vi "FuncImg-Extract selected ROIs data-Core.vi"(9 "System Cluster":T7 {"ROI number" min=1 format="ROI %.0f"}, 10 "Input cluster":T3={"Channel A?"=FALSE, "MovCor enabled"=FALSE, "Cycle time-stamps (us)"=[], "Cycle length (us)"=0.0, "[Pixels in ROI]"=[], "Z-Stack Header data"={"Number of POI"=0, "Number of Miniscans"=0, "Number of Trials"=0, "Number of Cycles "=0, "# Averaged Frames"=0, "Laser power (%)"=0, "Pockels"=0.0, "Acquisition Length (sec)"=0.0, "Fill time (us)"=0.0, "DwellTime (us)"=0.0, "Miniscan Dwell time per pixel (us)"=0.0, "PMT 1"=0.0, "PMT 2"=0.0, "Back Apperture"=0.0, "Zoom"=0.0, "Number of Pixels in Miniscan"=0, "Frame Size"=200, "Field of View"=0.0, "X centre"=0.0, "Y centre"=0.0, "AOL Z"=0.0}, "[ROI Time (us)]"=[], "Path out"=path "", "Version index"=0} {"Z-Stack Header data"."Frame Size" items=["100X100"=100, "128X128"=128, "200X200"=200, "256X256"=256, "512X512"=512, "1024x1024"=1024, "2048x2048"=2048]; "Z-Stack Header data"."Back Apperture" format="%#.6g"; "Z-Stack Header data"."Pockels" format="%#.6g"; "Z-Stack Header data"."PMT 2" format="%#.6g"; "Z-Stack Header data"."PMT 1" format="%#.6g"; "Z-Stack Header data"."Miniscan Dwell time per pixel (us)" format="%#.6g"; "Z-Stack Header data"."Zoom" format="%#.6g"; "Z-Stack Header data"."DwellTime (us)" format="%#.6g"; "Z-Stack Header data"."Acquisition Length (sec)" format="%#.6g"; "Z-Stack Header data"."Fill time (us)" format="%#.6g"}) -> (0 "error IO":errorcluster, 1 "Points per trial":i32, 3 "Interface-Data format definition":T4)   [LabVIEW 2017]
uses:
  xcontrol/Interface VIs/Interface typedefs/Interface-ROI selection cluster.ctl
  Typedefs/ROI ID Enum.ctl
  xcontrol/Interface VIs/Interface typedefs/Interface-Data format definition.ctl
  xcontrol/Typedefs/Xctl-XY data type definition.ctl
  xcontrol/Typedefs/Xctrl-ROI type enum.ctl
  Experiment header interface/Typedefs/Header parameters cluster-Zstack.ctl
  Typedefs/Frame Size.ctl
  xcontrol/XGrapher.xctl
panel:
  # "<--- Timeline data already decimated\n          for memory efficiency."
  # "Zstack header parameters"
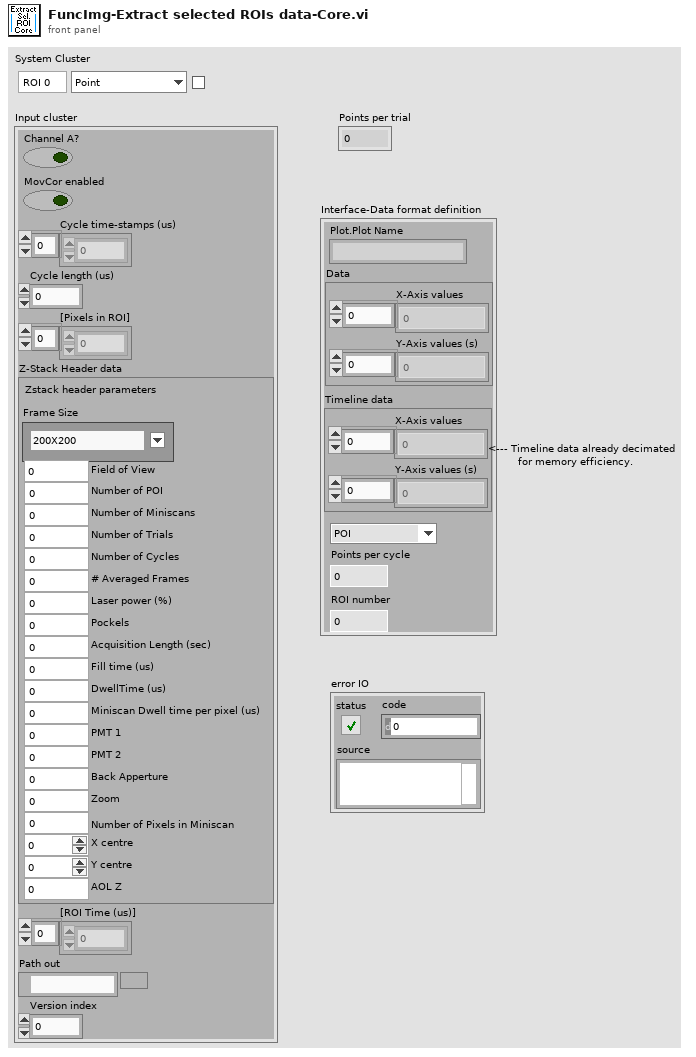
[diagram p1: front panel]
types:
  T1 = typedef "Header parameters cluster-Zstack.ctl" = cluster{"Number of POI":u16, "Number of Miniscans":u16, "Number of Trials":u16, "Number of Cycles ":u16, "# Averaged Frames":u16, "Laser power (%)":u8, "Pockels":dbl, "Acquisition Length (sec)":dbl, "Fill time (us)":dbl, "DwellTime (us)":dbl, "Miniscan Dwell time per pixel (us)":dbl, "PMT 1":dbl, "PMT 2":dbl, "Back Apperture":dbl, "Zoom":dbl, "Number of Pixels in Miniscan":u16, "Frame Size":T2, "Field of View":dbl, "X centre":dbl, "Y centre":dbl, "AOL Z":dbl}
  T2 = typedef "Frame Size.ctl" = u16
  T3 = cluster{"Channel A?":bool, "MovCor enabled":bool, "Cycle time-stamps (us)":dbl[], "Cycle length (us)":dbl, "[Pixels in ROI]":i32[], "Z-Stack Header data":T1, "[ROI Time (us)]":dbl[], "Path out":path, "Version index":i32}
  T4 = typedef "Interface-Data format definition.ctl" = cluster{"Plot.Plot Name":string, "Data":T5, "Timeline data":T5, "Type":T6, "Points per cycle":u16, "ROI number":u16}
  T5 = typedef "XGrapher.xctl/Xctl-XY data type definition.ctl" = cluster{"X-Axis values":sgl[], "Y-Axis values (s)":sgl[]}
  T6 = typedef "Xctrl-ROI type enum.ctl" = enum16{"POI", "Mini-scan", "Group"}
  T7 = typedef "Interface-ROI selection cluster.ctl" = cluster{"ROI number":i32, "ROI ID":T8, "Visibility":bool}
  T8 = typedef "ROI ID Enum.ctl" = enum16{"Point", "MiniScan", "Comp. MiniScan", "Rectangle", "Comp. volume", "Arb. plane point"}
  T9 = typedef "Interface-ROI type enum.ctl" = enum16{"POI", "Mini-scan"}
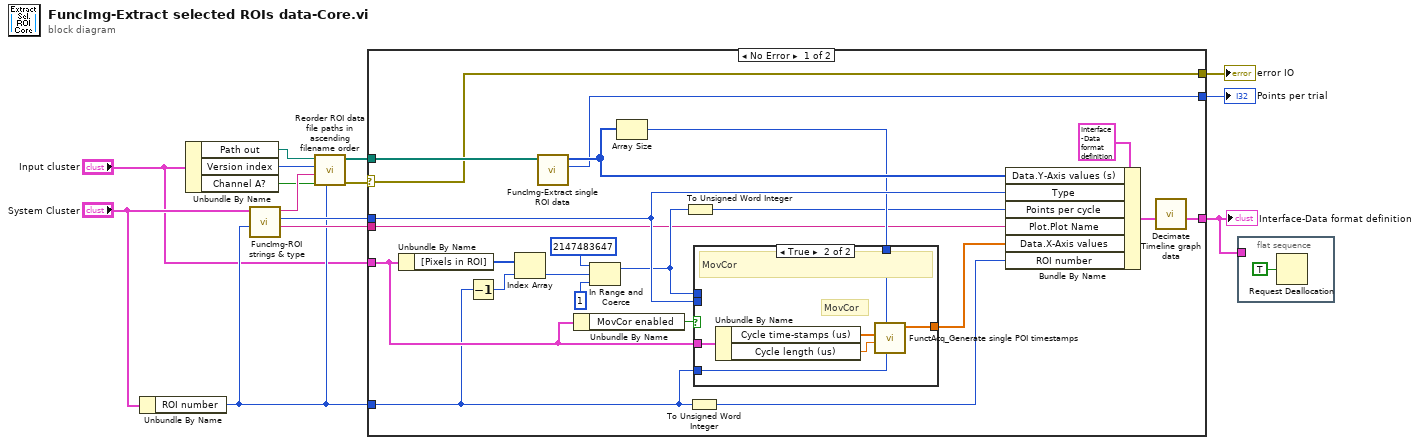
[diagram p0: block diagram]
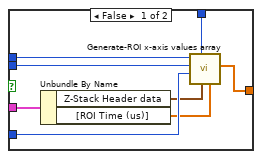
[diagram p2: hidden frame]
diagram:
  n1 = Unbundle By Name("System Cluster") -> ("ROI number"=w6:i32)
  n2 = Unbundle By Name("Input cluster") -> ("Path out"=w13:path, "Version index"=w14:i32, "Channel A?"=w10:bool)
  n3 = call "FuncImg-ROI strings & type.vi"("ROI number"=w6, "ROI visibility cluster"="System Cluster") -> ("Plot name"=w9:string, "ROI type"=w12:T9, "ROI ID string"=w11:string)  [unwired: 7 in]
  n4 = call "Reorder ROI data file paths in ascending filename order.vi"("ROI number"=w6, "Channel A?"=w10, "ROI ID string"=w11, "ROI file format version"=w14, "Dataset directory path"=w13) -> ("Error out"=w4:errorcluster, "Reordered file paths in ascending file-name order"=w2:path[])  [unwired: 5 in]
  n5 = case shown="No Error" w4 {
    selector: w4 -> [w17 w51]
    tunnel: w12 -> [w34 _]
    tunnel: w2 -> [w32 _]
    tunnel: w9 -> [w22 _]
    tunnel: [w21 _] -> w8
    tunnel: w6 -> [w15 _]
    tunnel: "Input cluster" -> [w16 _]
    tunnel: [w18 _] -> w1
    tunnel: [w17 w51] -> w3
    frame No Error {
      n6 = Unbundle By Name(w16) -> ("[Pixels in ROI]"=w35:i32[])
      n7 = Decrement(x=w15) -> (x-1=w29:i32)
      n8 = Index Array(array=w35, index=w29) -> (element=w23:i32)
      n9 = call "FuncImg-Extract single ROI data.vi"("Reordered file paths in ascending file-name order"=w32) -> ("Points per trial"=w21:i32, "Data. Y-Axis values"=w33:i32[])  [unwired: 9 in]
      n10 = Unbundle By Name(w16) -> ("MovCor enabled"=w36:bool)
      n11 = In Range and Coerce(upper limit=2147483647, x=w23, lower limit=1) -> (coerced(x)=w27:i32)  [unwired: 1 out]
      n12 = Array Size(array=w33) -> (size(s)=w30:i32)
      n13 = To Unsigned Word Integer(number=w27) -> (unsigned 16bit integer=w26:u16)
      n14 = To Unsigned Word Integer(number=w15) -> (unsigned 16bit integer=w28:u16)
      n15 = case shown="True" w36 {
        tunnel: w34 -> [w44 _]
        tunnel: w27 -> [w43 _]
        tunnel: w15 -> [w42 w49]
        tunnel: w30 -> [w41 w50]
        tunnel: [w40 w48] -> w20
        tunnel: w16 -> [w39 w45]
        frame False {
          n16 = Unbundle By Name(w39) -> ("Z-Stack Header data"=w38:T1, "[ROI Time (us)]"=w37:dbl[])
          n17 = call "Generate-ROI x-axis values array.vi"("[ROI Time(us)]"=w37, "Header data"=w38, "Number of points in Y-axis array"=w41, "ROI number"=w42, "Type"=w44, "Pixels in ROI"=w43) -> ("ROI X-axis values array (sec)"=w40:sgl[])  [unwired: 5 in]
        }
        frame True {
          # "MovCor"
          # "MovCor"
          n18 = Unbundle By Name(w45) -> ("Cycle time-stamps (us)"=w47:dbl[], "Cycle length (us)"=w46:dbl)
          n19 = call "FunctAcq_Generate single POI timestamps.vi"("ROI number"=w49, "Number of data points in single POI (all trials)"=w50, "Funct Acq cycle length (us)"=w46, "Single funct.acq cycle time-stamps (us)"=w47) -> ("Full timestamps array for single POI (sec)"=w48:sgl[])  [unwired: 7 in]
        }
      }
      n20 = Bundle By Name(cluster=T4 {"Plot.Plot Name"="", "Data"={"X-Axis values"=[], "Y-Axis values (s)"=[]}, "Timeline data"={"X-Axis values"=[], "Y-Axis values (s)"=[]}, "Type"=enum."POI", "Points per cycle"=0, "ROI number"=0}, "Data.Y-Axis values (s)"=w33, "Type"=w34, "Points per cycle"=w26, "Plot.Plot Name"=w22, "Data.X-Axis values"=w20, "ROI number"=w28) -> (w19:T4)
      n21 = call "Decimate Timeline graph data.vi"("Data in"=w19) -> ("Data out"=w18:T4)  [unwired: 10 in]
    }
    frame Error {
    }
  }
  "Interface-Data format definition" <- w1
  "Points per trial" <- w8
  "error IO" <- w3
  n22 = flat-sequence {
    tunnel: w1 -> [_]
    frame #0 {
      n23 = Request Deallocation(TRUE ("flag")) -> ()
    }
  }
